vi "P3.5.vi"() -> ()   [LabVIEW 2020]
uses:
  <vilib>/Analysis/2dsp.llb/Real FFT.vi
  <vilib>/Analysis/NI_AALPro.lvlib
panel:
  out "FFT manual 32":dbl[](graph)
  out "FFT manual 16":dbl[](graph)
  out "Señal original":dbl[](graph)
  out "Señal + 0s":dbl[](graph)
  out "Señal 128":dbl[](graph)
  out "Size X128":i32
  out "Size X32":i32
  out "Size X16":i32
  out "Señal 32":dbl[](graph)
  out "Señal 16":dbl[](graph)
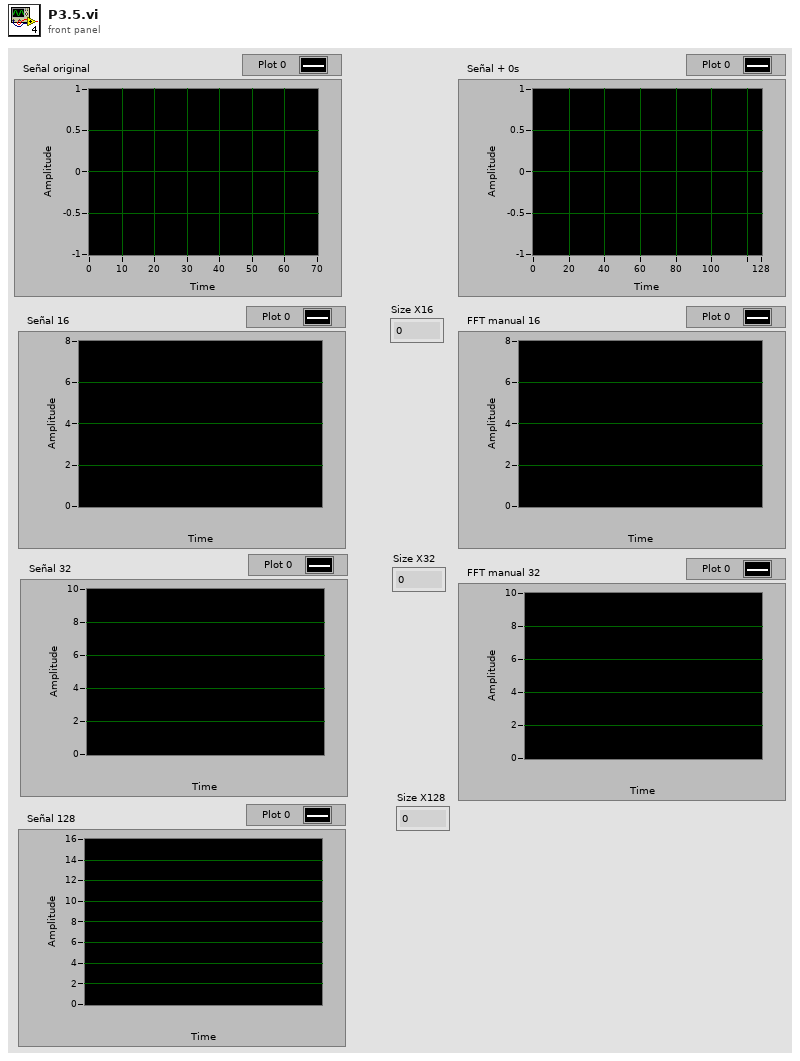
[diagram p1: front panel]
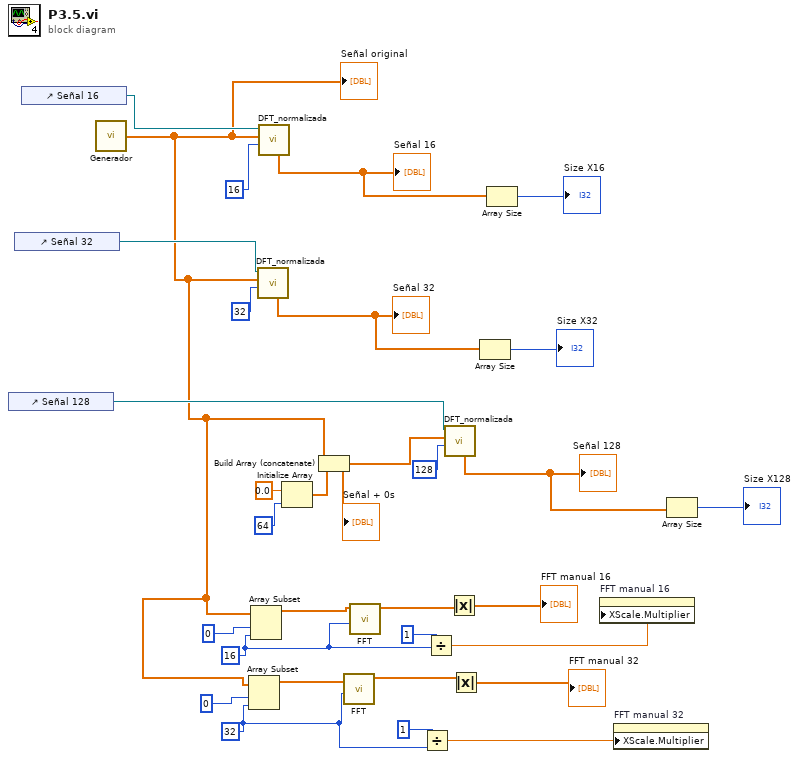
[diagram p0: block diagram]
diagram:
  w10 = 32 ("length")
  w12 = 16 ("length")
  n1 = control-ref of="Señal 128"() -> (w23:refnum<vi>)
  n2 = control-ref of="Señal 32"() -> (w30:refnum<vi>)
  n3 = control-ref of="Señal 16"() -> (w31:refnum<vi>)
  n4 = call "Generador.vi"() -> ("Signal"=w16:dbl[])  [unwired: 1 in]
  "Señal original" <- w16
  n5 = Array Subset(array=w16, index=0, length=w10) -> (w14:dbl[])
  n6 = Array Subset(array=w16, index=0, length=w12) -> (w15:dbl[])
  n7 = call "DFT_normalizada.vi"("FFT size"=32, "X[n]"=w16, "WaveformGraph in"=w30) -> ("SubX"=w7:cdb[])  [unwired: 8 in]
  "Señal 32" <- w7
  n8 = call "DFT_normalizada.vi"("FFT size"=16, "X[n]"=w16, "WaveformGraph in"=w31) -> ("SubX"=w8:cdb[])  [unwired: 8 in]
  "Señal 16" <- w8
  n9 = Initialize Array(0.0 ("element"), 64 ("dimension size")) -> (w20:dbl[])
  n10 = Build Array (concatenate)(w16, w20) -> (w19:dbl[])
  "Señal + 0s" <- w19
  n11 = call-poly <vilib>:"FFT.vi"("FFT size"=w10, "X"=w14) -> ("FFT {X}"=w3:cdb[])  [unwired: 8 in, 1 out]
  n12 = call-poly <vilib>:"FFT.vi"("FFT size"=w12, "X"=w15) -> ("FFT {X}"=w5:cdb[])  [unwired: 8 in, 1 out]
  n13 = Divide(x=1, y=w10) -> (x/y=w9:dbl)
  n14 = Divide(x=1, y=w12) -> (x/y=w4:dbl)
  n15 = call "DFT_normalizada.vi"("FFT size"=128, "X[n]"=w19, "WaveformGraph in"=w23) -> ("SubX"=w6:cdb[])  [unwired: 8 in]
  "Señal 128" <- w6
  n16 = Absolute Value(x=w5) -> (abs(x)=→"FFT manual 16":dbl[])
  n17 = Absolute Value(x=w3) -> (abs(x)=→"FFT manual 32":dbl[])
  n18 = Array Size(array=w7) -> (size(s)=→"Size X32":i32)
  n19 = Array Size(array=w8) -> (size(s)=→"Size X16":i32)
  n20 = property on="FFT manual 16" class="WFGraph (strict)"("XScale.Multiplier"=w4) -> ()  [unwired: 2 in, 2 out]
  n21 = property on="FFT manual 32" class="WFGraph (strict)"("XScale.Multiplier"=w9) -> ()  [unwired: 2 in, 2 out]
  n22 = Array Size(array=w6) -> (size(s)=→"Size X128":i32)
